vi "Read Path.vi"(8 "error in (no error)":errorcluster, 9 "Default If Not Found":path, 10 "Name":string, 11 "IConfiguration in":refnum<class "IConfiguration.lvclass">) -> (0 "error out":errorcluster, 1 "Not Found?":bool, 2 "Value":path, 3 "IConfiguration out":refnum<class "IConfiguration.lvclass">)   [LabVIEW 2017, in "Configuration.lvlib" / "IConfiguration.lvclass"]
uses:
  IConfiguration.lvclass
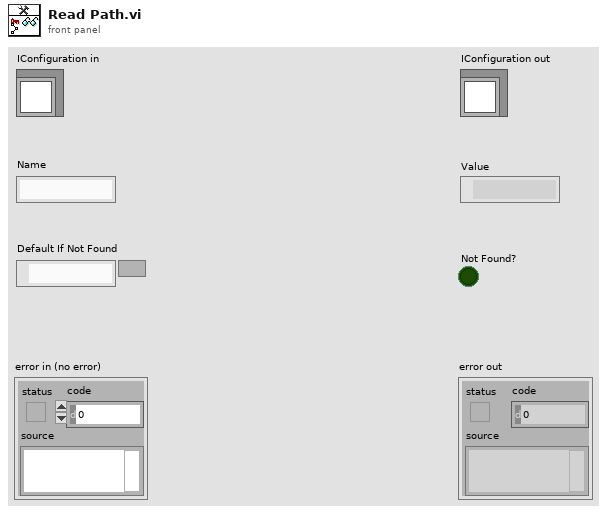
[diagram p1: front panel]
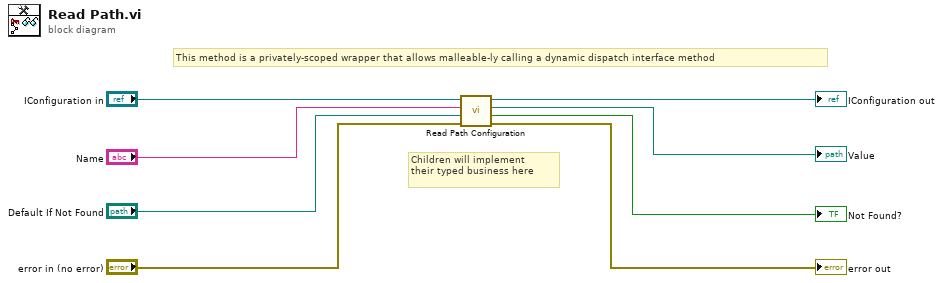
[diagram p0: block diagram]
diagram:
  # "Children will implement\ntheir typed business here"
  # "This method is a privately-scoped wrapper that allows malleable-ly calling a dynamic dispatch interface method"
  n1 = call-dynamic "Read Path Configuration.vi"("error in (no error)"="error in (no error)", "Default If Not Found"="Default If Not Found", "Name"="Name", "IConfiguration in"="IConfiguration in") -> ("error out"=→"error out":errorcluster, "Not Found?"=→"Not Found?":bool, "Value"=→"Value":path, "IConfiguration out"=→"IConfiguration out":refnum<class "IConfiguration.lvclass">)  [unwired: 4 in]
